vi "Global.vi"() -> ()   [LabVIEW 2012, in "AIT 429 Custom Device.lvlib"]
uses:
  AIT 429 Custom Device.lvlib
panel:
  in  "Timestamp Channel GUID (default)":string="03D3BB99-1485-13A6-561D1F898F032919"
  in  "bufferSize":string="bufferSize"
  in  "TransferType":string="TransferType"
  in  "Word Section Page GUID":string="e863b59a-2425-4ba9-866f-b01b318941b7"
  in  "Specify module by":string="Specify module by"
  in  "ScheduledSDI":string="ScheduledSDI"
  in  "xmlName":string="xmlName"
  in  "SDIValue":string="SDIValue"
  in  "SDI_Enabled":string="SDI_Enabled"
  in  "ScaleOffset":string="ScaleOffset"
  in  "ScaleFac":string="ScaleFac"
  in  "Signed?":string="Signed?"
  in  "InBufferSize":string="InBufferSize"
  in  "txRate":string="txRate"
  in  "DBHash":string="DBHash"
  in  "WinBinCache":string="Temp429BinFiles"
  in  "MainDisabled":string="C84F327B-5F00-A71A-4A47-A7C0FE0BF79D"
  in  "MainEnabled":string="961BA415-D612-25DB-1EE4-93AC9399C9B8"
  in  "InputsReadRate":string="InputsReadRate"
  in  "InLoopTime":string="Inputs Loop Duration"
  in  "OutLoopTime":string="Outputs Loop Duration"
  in  "Status Section":string="Status"
  in  "Error Code":string="Error Code"
  in  "HWIn Late Count":string="Inputs Late Count"
  in  "HWOut Late Count":string="Outputs Late Count"
  in  "Static Chan GUID":string="620FF26C-B46F-A798-9FE7-99E7CBCC898B"
  in  "Default word":string="Default word"
  in  "Module#":string="Module#"
  in  "Status Section GUID":string="40A8AAAE-6936-1961-F317-B9DADC611A49"
  in  "Num Bits":string="Num Bits"
  in  "Channel Page GUID":string="7E8619EB-70E6-9299-14EE-99E8B20A7109"
  in  "Channel #":string="Channel #"
  in  "HWOutputs GUID":string="B316C0B3-A1A3-75D9-9053-C890A1BD32E0"
  in  "HWInputs GUID":string="3FB60206-0B92-B78E-8988-3E4A690C747C"
  in  "Win File Path":string="Win File Path"
  in  "Start Bit":string="Start Bit"
  in  "RT File Path":string="RT File Path"
  in  "Type":string="Type"
  in  "Outputs":string="Outputs"
  in  "Inputs":string="Inputs"
  in  "transferPeriod":string="transferPeriod"
  in  "Label Section Page GUID":string="961BA415-D612-25DB-1EE4-93AC9399C911"
  in  "Label Data Page GUID":string="961BA415-D612-25DB-1EE4-93AC9399C951"
  in  "Label":string="Label"
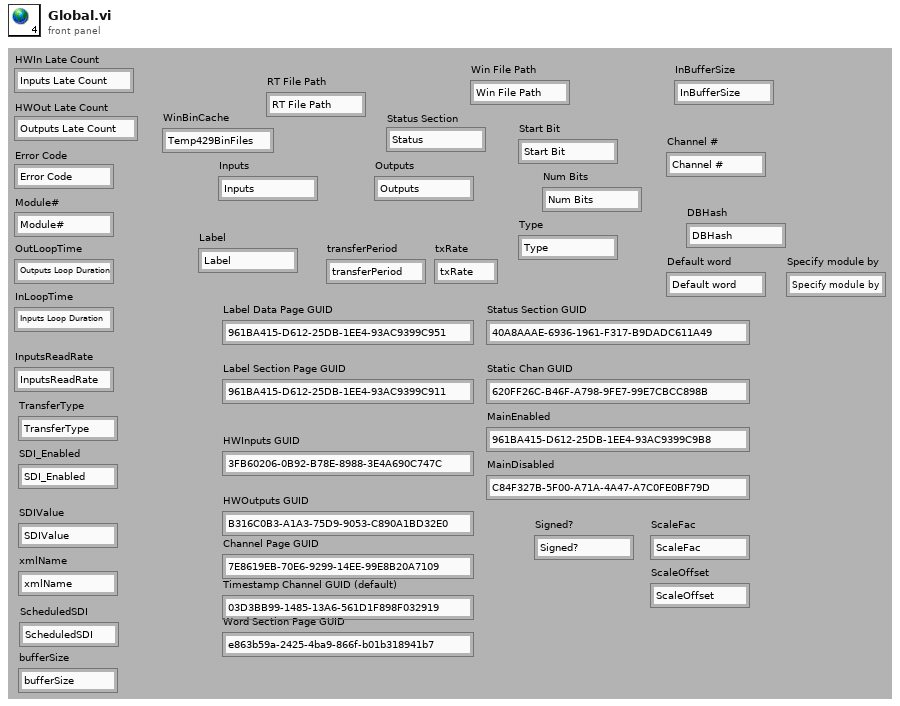
[diagram p1: front panel]
diagram:
